vi "Wideband Spectrum Analyser.vi"(7 "Averaging Parameters":T1={"averaging mode"=enum."RMS averaging", "weighting mode"=enum."Linear", "number of averages"=10} {"number of averages" min=1}, 9 "Display Settings":cluster{"display unit":u16, "log/linear":u16}={"display unit"=2, "log/linear"=2} {"log/linear" items=["Linear", "dB", "dBm"]; "display unit" items=["Vrms", "Vpk", "Vrms^2", "Vpk^2", "Vrms/rtHz", "Vpk/rtHz", "Vrms^2/Hz", "Vpk^2/Hz"]}, 10 "Rx Parameters":T2={"IQ Sampling\nRate [S/sec]"=1000000.0, "Acq Duration [sec]"=0.001, "Start Carrier [Hz]"=88000000.0, "Stop Carrier [Hz]"=108000000.0, "Gain [dB]"=25.0, "Active Antenna"="RX2", "Reference Source"="Internal", "Timebase Source"="Internal"} {"Gain [dB]" format="%#_4g"; "Stop Carrier [Hz]" min=50000000.0 max=6000000000.0 step=1000.0 format="%#.15p"; "Start Carrier [Hz]" min=50000000.0 max=6000000000.0 step=1000.0 format="%#.15p"; "Acq Duration [sec]" min=0.0 step=0.001 format="%#.6p"; "IQ Sampling\nRate [S/sec]" format="%#_6p"}, 11 "USRP IP Address":refnum<k15>="192.168.12.4") -> (0 "error out":errorcluster, 2 "FFT Power Spectrum":cluster{"f0":dbl, "df":dbl, "IQ":dbl[]}(graph)={"f0"=87750000.0, "df"=1000.0, "IQ"=array[20500 elements]})   [LabVIEW 2017]
panel:
  in  "Dynamic Range (dB)":cluster{dbl, dbl}(slide)={0.09852216748768905, -121.37931034482759} scale=-140.0..40.0
  in  "Waterfall Time Scale (s)":i32=5
  out "Waterfall Plot":dbl[][](graph)
  out "Loop Counter":i32
  in  "STOP RECORDING":bool
  in  "stop":bool
  # "Wideband Spectrum (Averaged)"
  # "Graph Controls"
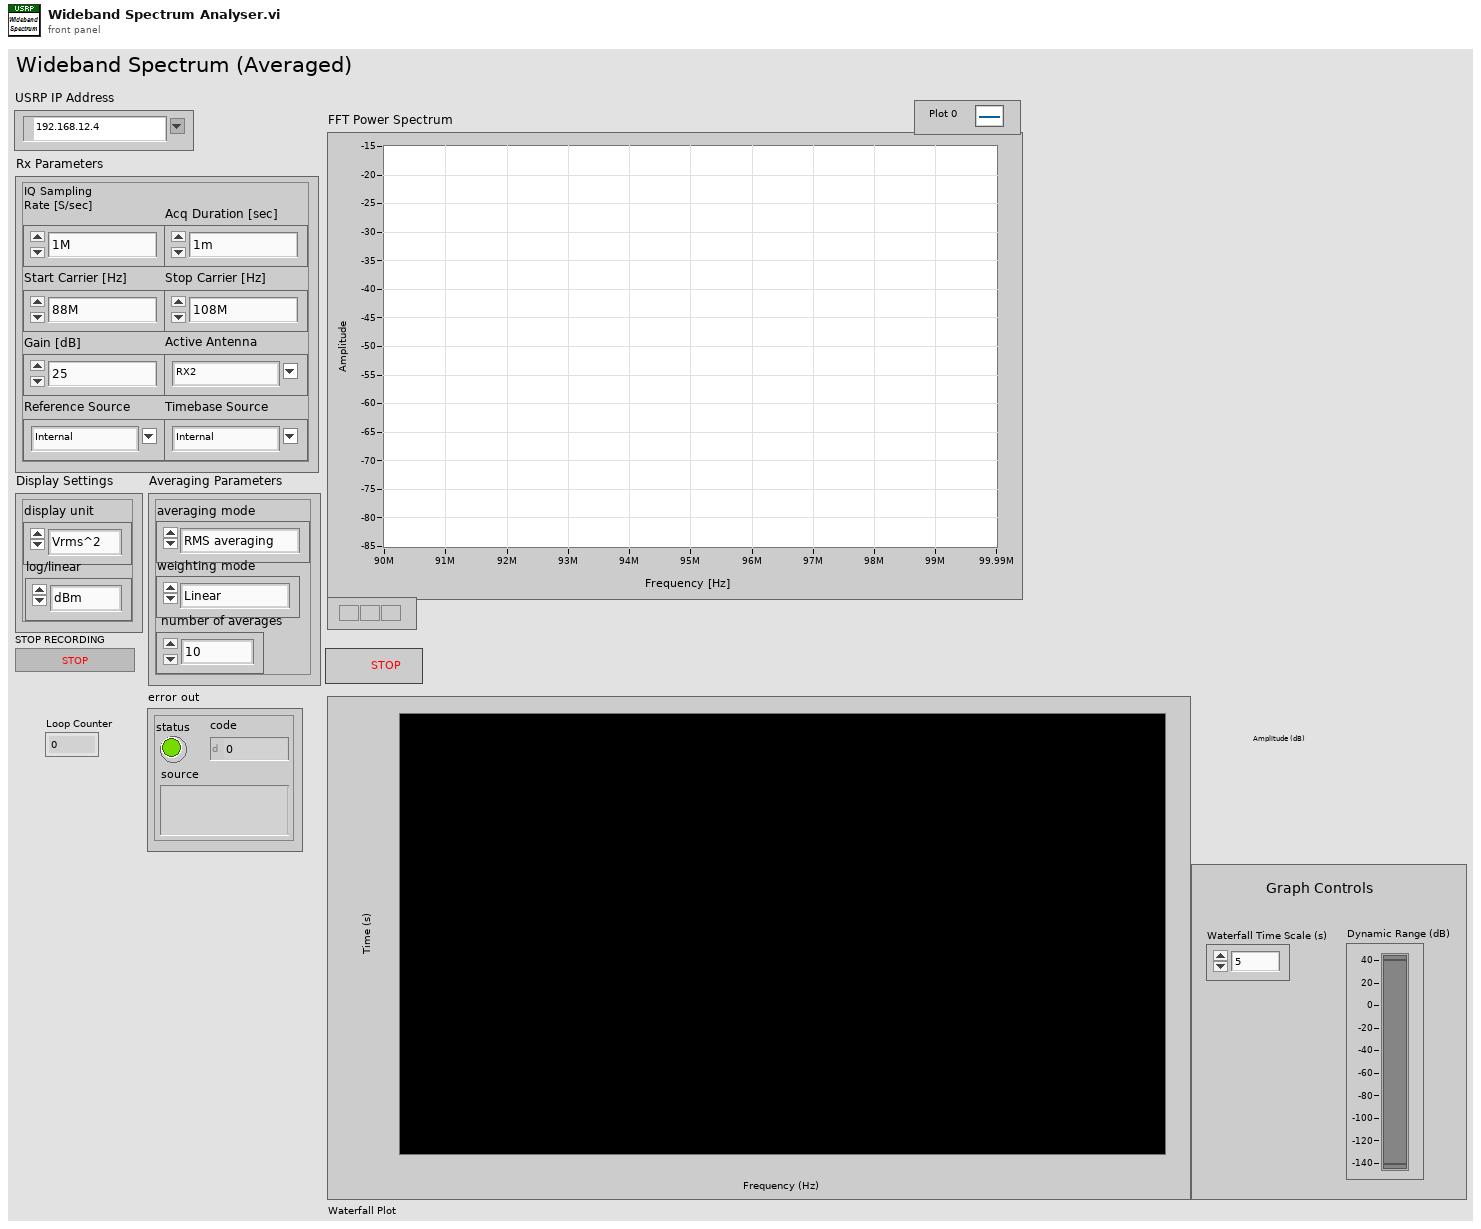
[diagram p1: front panel]
types:
  T1 = cluster{"averaging mode":enum16{"No averaging", "Vector averaging", "RMS averaging", "Peak hold"}, "weighting mode":enum16{"Linear", "Exponential"}, "number of averages":u32}
  T2 = cluster{"IQ Sampling\nRate [S/sec]":dbl, "Acq Duration [sec]":dbl, "Start Carrier [Hz]":dbl, "Stop Carrier [Hz]":dbl, "Gain [dB]":dbl, "Active Antenna":string, "Reference Source":string, "Timebase Source":string}
  T3 = typedef "subFrameParams.ctl" = cluster{"IQ Rate":dbl, "Frames":i32, "Length of Subset":i32, "Start Index of Subset":i32, "Start Carrier [Hz]":dbl, "Stop Carrier [Hz]":dbl, "Acq Duration [sec]":dbl}
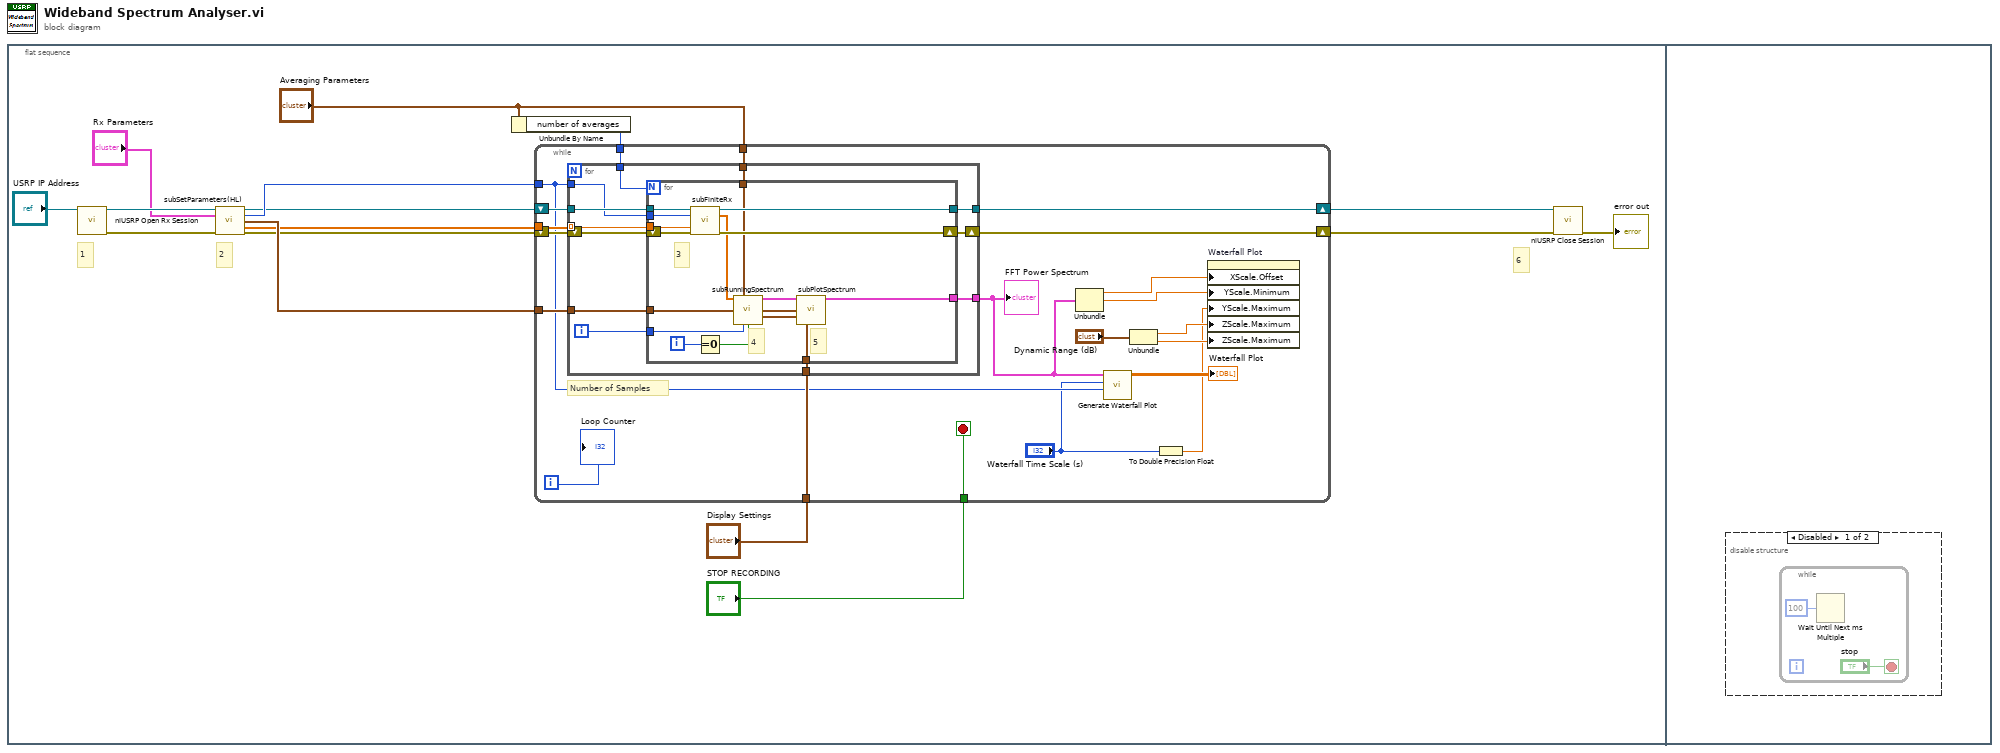
[diagram p0: block diagram]
diagram:
  n1 = flat-sequence {
    frame #0 {
      # "6"
      # "2"
      # "1"
      n2 = call <instrlib>:"niUSRP Open Rx Session.vi"("device names"="USRP IP Address") -> ("session handle out"=w11:refnum<k15>, "error out"=w10:errorcluster)  [unwired: 13 in]
      n3 = call "subSetParameters(HL).vi"("IVI Refnum in"=w11, "Rx Parameters"="Rx Parameters", "error in (no error)"=w10) -> ("IVI Refnum out"=w3:refnum<k15>, "samples per acquisition"=w13:i32, "Frame Parameters"=w8:T3, "test carrier frequencies"=w7:dbl[], "error out"=w2:errorcluster)  [unwired: 8 in]
      n4 = Unbundle By Name("Averaging Parameters") -> ("number of averages"=w5:u32)
      n5 = while {
        tunnel: w13 -> [w26]
        tunnel: w8 -> [w35]
        tunnel: w7 -> [w34]
        tunnel: "Display Settings" -> [w33]
        tunnel: w5 -> [w32]
        tunnel: "Averaging Parameters" -> [w31]
        shift-right: [w37] -> w15
        shift-left: w3 -> [w30]
        shift-right: [w36] -> w14
        shift-left: w2 -> [w29]
        tunnel: "STOP RECORDING" -> [w28]
        i -> [w27]
        stop <- w28 stop-if-true
        # "Number of Samples"
        n6 = for {
          tunnel: w30 -> [w49]
          tunnel: w26 -> [w43]
          tunnel: [w48] -> w37
          shift-right: [w42] -> w36
          shift-left: w29 -> [w47]
          tunnel: w35 -> [w46]
          tunnel: w34 -> [w45] mode=indexing
          tunnel: w33 -> [w44]
          tunnel: w32 -> [w41]
          tunnel: w31 -> [w40]
          tunnel: [w38] -> w24
          i -> [w39]
          n7 = for {
            N: w41 -> [_]
            tunnel: w49 -> [w66]
            tunnel: [w65] -> w48
            tunnel: w39 -> [w64]
            tunnel: w46 -> [w61]
            tunnel: w45 -> [w60]
            tunnel: w44 -> [w57]
            tunnel: w43 -> [w56]
            shift-right: [w55] -> w42
            shift-left: w47 -> [w63]
            tunnel: w40 -> [w54]
            tunnel: [w50] -> w38
            i -> [w52]
            # "5"
            # "4"
            # "3"
            n8 = call "subFiniteRx.vi"("IVI Refnum in"=w66, "Number of Samples"=w56, "Carrier Frequency"=w60, "error in (no error)"=w63) -> ("IVI Refnum out"=w65:refnum<k15>, "data"=w51:cdb[], "error out"=w55:errorcluster)  [unwired: 9 in]
            n9 = Equal To 0?(x=w52) -> (x = 0?=w53:bool)
            n10 = call "subRunningSpectrum.vi"("Input Baseband IQ"=w51, "averaging parameters"=w54, "restart averaging"=w53, "Frame Parameters"=w61, "Iteration"=w64) -> ("Spectrum to Plot"=w62:cluster{"f0":dbl, "df":dbl, "IQ":dbl[]}, "Frame Parameters out"=w59:T3, "window properties"=w58:cluster{"eq noise BW":dbl, "coherent gain":dbl})  [unwired: 7 in, 1 out]
            n11 = call "subPlotSpectrum.vi"("Spectrum to Plot"=w62, "Frame Parameters"=w59, "window properties"=w58, "Display"=w57) -> ("Spectrum to Plot"=w50:cluster{"f0":dbl, "df":dbl, "IQ":dbl[]})  [unwired: 11 in]
          }
        }
        "FFT Power Spectrum" <- w24
        n12 = Unbundle(w24) -> ("f0"=w20:dbl, "df"=w19:dbl)  [unwired: 1 out]
        n13 = call "Generate Waterfall Plot.vi"("number of samples"=w26, "Waterfall Time Scale (s)"="Waterfall Time Scale (s)", "power spectrum"=w24) -> ("Waterfall Plot Output"=→"Waterfall Plot":dbl[][])  [unwired: 8 in]
        n14 = Unbundle("Dynamic Range (dB)") -> (w21:dbl, w22:dbl)
        n15 = To Double Precision Float(number="Waterfall Time Scale (s)") -> (double precision float=w17:dbl)
        n16 = property on="Waterfall Plot" class="IntGraph (strict)"("XScale.Offset"=w20, "YScale.Minimum"=w19, "YScale.Maximum"=w17, "ZScale.Maximum"=w21, "ZScale.Maximum"=w22) -> ()  [unwired: 2 in, 2 out]
        "Loop Counter" <- w27
      }
      n17 = call <instrlib>:"niUSRP Close Session.vi"("session handle"=w15, "error in (no error)"=w14) -> ("error out"=→"error out":errorcluster)  [unwired: 13 in]
    }
    frame #1 {
      n18 = disable-structure shown="Disabled" {
        frame Disabled {
          n19 = while {
            stop <- "stop" stop-if-true
            n20 = Wait Until Next ms Multiple(millisecond multiple=u32 100) -> ()  [unwired: 1 out]
          }
        }
        frame Enabled {
        }
      }
    }
  }
